vi "bt_test3_struct_data.vi"() -> ()   [LabVIEW 2025]
panel:
  in  "VI Path":string
  in  "Send Alarm":bool
  in  "Alarm Type":string
  in  "Alarm Temperature":dbl
  in  "Alarm Time":string
  in  "Normal Temperature":dbl
  in  "Send Normal":bool
  out "String":string
  out "BT Status":bool
  in  "BT Switch":bool
  out "error out":errorcluster
  in  "stop":bool
  in  "Python Script Path":path
  in  "Python Interpreter Path":path
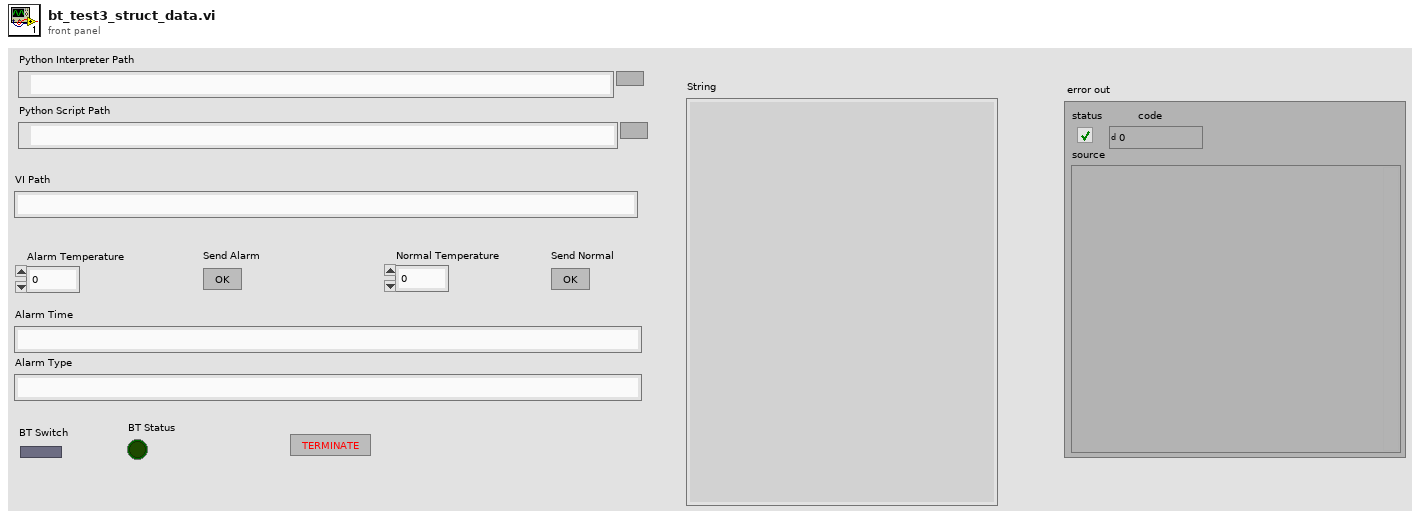
[diagram p1: front panel]
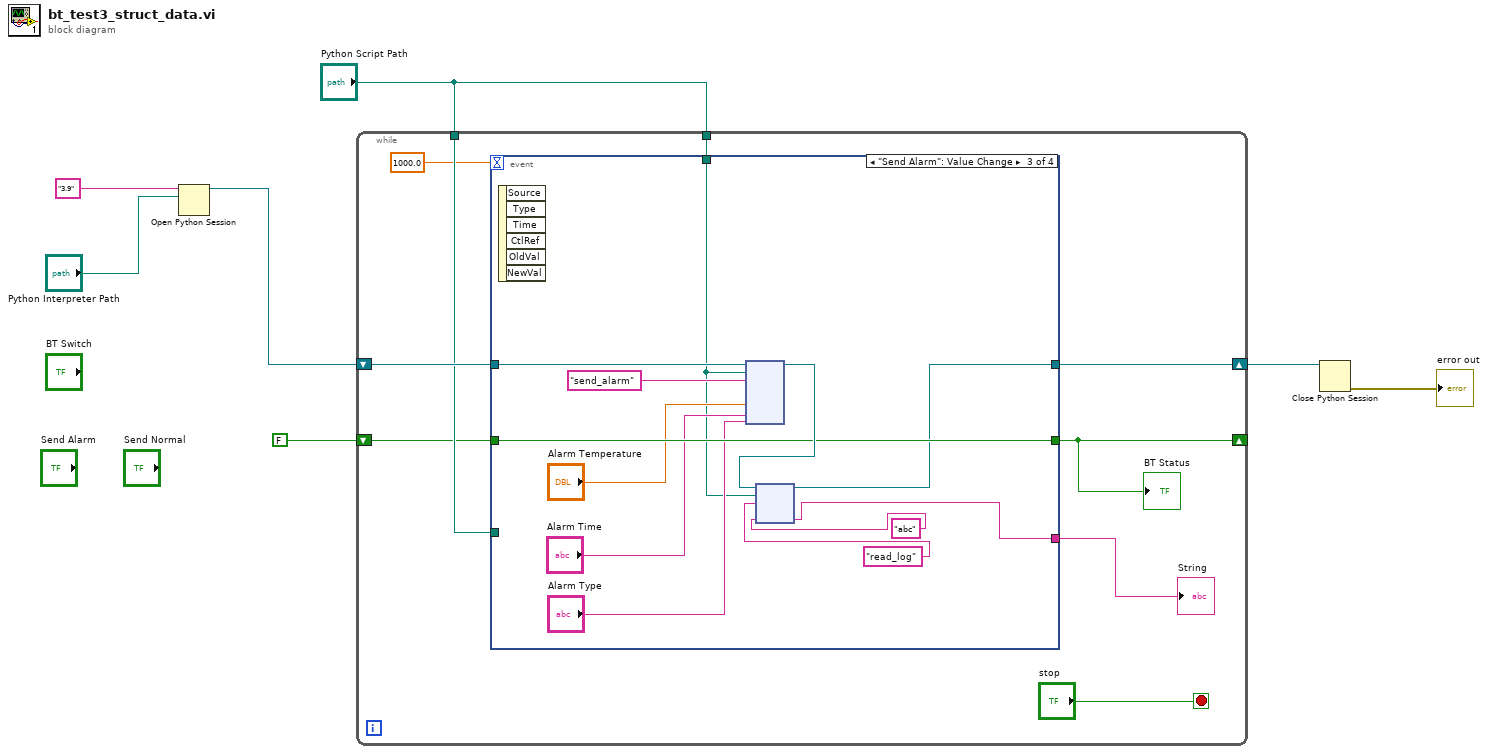
[diagram p0: block diagram]
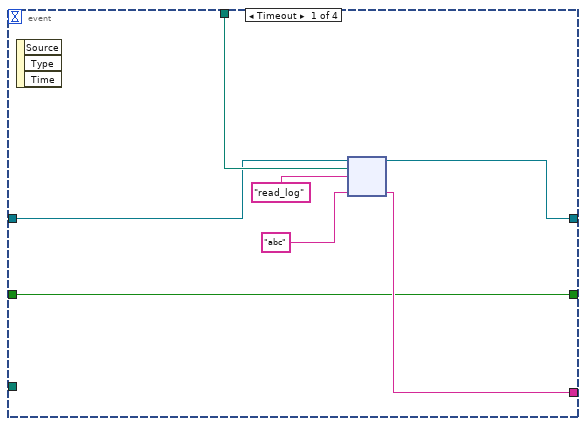
[diagram p2: hidden frame]
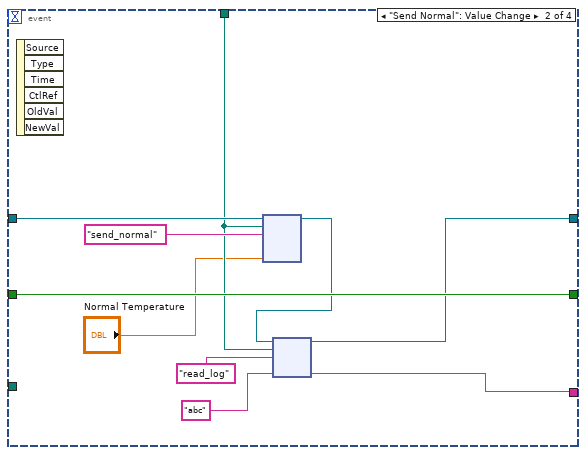
[diagram p3: hidden frame]
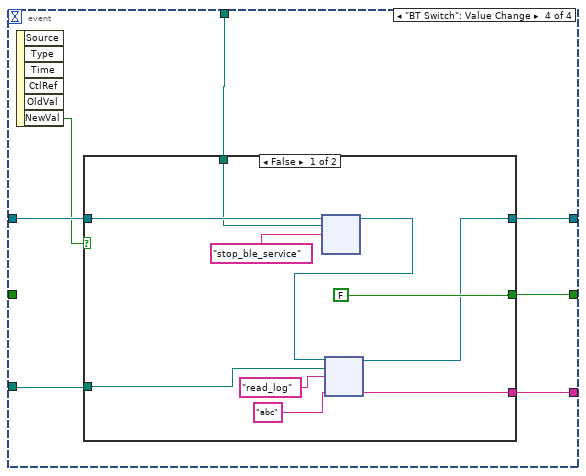
[diagram p4: hidden frame]
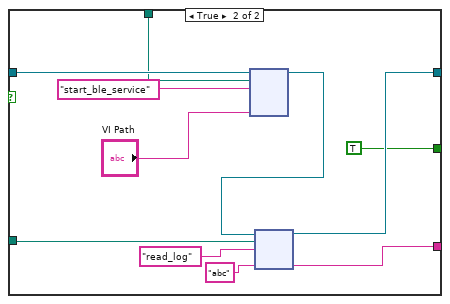
[diagram p5: hidden frame]
diagram:
  n1 = Open Python Session(python version="3.9", python path="Python Interpreter Path") -> (session out=w5:refnum<k35>)  [unwired: 1 in, 1 out]
  n2 = while {
    shift-right: [w12] -> w2
    shift-left: w5 -> [w15]
    shift-right: [w8] -> _
    shift-left: FALSE -> [w9]
    tunnel: "Python Script Path" -> [w14]
    tunnel: "Python Script Path" -> [w13]
    stop <- "stop" stop-if-true
    n3 = event shown="[2] \"Send Alarm\": Value Change" {
      selector: _ -> [_ _ _ _]
      dyn-events: _ -> [_ _ _ _]
      timeout: 1000.0 -> [_ _ _ _]
      tunnel: w15 -> [w21 w32 w40 w52]
      tunnel: [w20 w26 w39 w51] -> w12
      tunnel: w14 -> [w22 w25 w35 w50]
      tunnel: w13 -> [_ _ _ w49]
      tunnel: [w18 w28 w34 w48] -> w11
      tunnel: w9 -> [w17 w31 w41 _]
      tunnel: [w17 w31 w41 w46] -> w8
      event Timeout {
        n4 = event-data() -> ()  [unwired: 1 in, 3 out]
        n5 = node(w21, w22, "read_log", "abc") -> (w20:refnum<k35>, w18:string)  [unwired: 1 in, 3 out]
      }
      event "Send Normal": Value Change {
        n6 = event-data() -> ()  [unwired: 1 in, 6 out]
        n7 = node(w32, w25, "send_normal", "Normal Temperature") -> (w27:refnum<k35>)  [unwired: 4 in, 3 out]
        n8 = node(w27, w25, "read_log", "abc") -> (w26:refnum<k35>, w28:string)  [unwired: 1 in, 3 out]
      }
      event "Send Alarm": Value Change {
        n9 = event-data() -> ()  [unwired: 1 in, 6 out]
        n10 = node(w40, w35, "send_alarm", "Alarm Temperature", "Alarm Time", "Alarm Type") -> (w45:refnum<k35>)  [unwired: 6 in, 3 out]
        n11 = node(w45, w35, "read_log", "abc") -> (w39:refnum<k35>, w34:string)  [unwired: 1 in, 3 out]
      }
      event "BT Switch": Value Change {
        n12 = event-data() -> ("NewVal"=w47:bool)  [unwired: 1 in, 5 out]
        n13 = case shown="False" w47 {
          tunnel: w52 -> [w61 w72]
          tunnel: [w57 w69] -> w51
          tunnel: [FALSE TRUE] -> w46
          tunnel: w50 -> [w55 w68]
          tunnel: w49 -> [w56 w67]
          tunnel: [w53 w64] -> w48
          frame False {
            n14 = node(w61, w55, "stop_ble_service") -> (w58:refnum<k35>)  [unwired: 3 in, 3 out]
            n15 = node(w58, w56, "read_log", "abc") -> (w57:refnum<k35>, w53:string)  [unwired: 1 in, 3 out]
          }
          frame True {
            n16 = node(w72, w68, "start_ble_service", "VI Path") -> (w70:refnum<k35>)  [unwired: 4 in, 3 out]
            n17 = node(w70, w67, "read_log", "abc") -> (w69:refnum<k35>, w64:string)  [unwired: 1 in, 3 out]
          }
        }
      }
    }
    "BT Status" <- w8
    "String" <- w11
  }
  n18 = Close Python Session(session in=w2) -> (11:→"error out":errorcluster)  [unwired: 1 in]
